vi "Global Number of Indices.vi"() -> ()   [LabVIEW 2020]
panel:
  in  "Number of indicies":u8
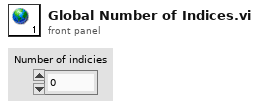
[diagram p1: front panel]
diagram:
